vi "databaseDirectory (SubVI).vi"() -> (0 "Application Directory":path)   [LabVIEW 2013]
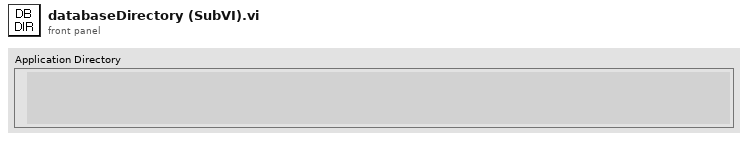
[diagram p1: front panel]
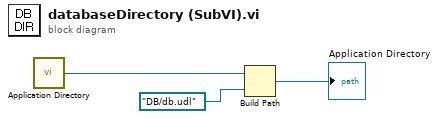
[diagram p0: block diagram]
diagram:
  n1 = call <vilib>:"Application Directory.vi"() -> ("Application Directory"=w2:path)
  n2 = Build Path(base path=w2, name or relative path=path "DB/db.udl" ("Application:Directory Path")) -> (appended path=→"Application Directory":path)
